vi "ADAM 5000 Get Data.vi"(11 "TCP Connection Refnum in":refnum<k5>) -> (1 "Voltages":dbl[](array[numeric])=[0.7972994999999994, -0.009129000000000609, -0.009129000000000609, -0.009585900000000258, -0.009129000000000609, -0.009585900000000258, -0.009585900000000258, -0.009585900000000258], 2 "TC Array":dbl[](array[numeric])=[21.380699999999997, 27.4835, 27.4835, 27.4835, 27.4835, 27.378999999999998, 27.4835], 3 "TCP Connection Refnum (dup)":refnum<k5>)   [LabVIEW 2018]
uses:
  nimodbus121/71/vi.lib/NI Modbus.llb/MB Modbus Command.ctl
panel:
  out "error out 2":errorcluster
  in  "Modbus Voltage Command":T1={"Function Code"=3, "Starting Address"=0, "Quantity"=8, "Data"=[], "Discrete"=[]} {"Function Code" items=["Read Coils"=1, "Read Discrete Inputs"=2, "Read Holding Registers"=3, "Read Input Registers"=4, "Write Single Coil"=5, "Write Single Register"=6, "Read Exception Status"=7, "Write Multiple Coils"=15, "Write Multiple Registers"=16]}
  out "Slave Input Registers 3":u16[](array[numeric])=[38065, 32770, 32770, 32767, 32770, 32767, 32767, 32767] caption="Slave Input Registers (Read Only)"
  out "error out":errorcluster
  in  "Modbus TC Command":T1={"Function Code"=3, "Starting Address"=16, "Quantity"=7, "Data"=[], "Discrete"=[]} {"Function Code" items=["Read Coils"=1, "Read Discrete Inputs"=2, "Read Holding Registers"=3, "Read Input Registers"=4, "Write Single Coil"=5, "Write Single Register"=6, "Read Exception Status"=7, "Write Multiple Coils"=15, "Write Multiple Registers"=16]}
  out "Slave Input Registers 2":u16[](array[numeric])=[1023, 1315, 1315, 1315, 1315, 1310, 1315] caption="Slave Input Registers (Read Only)"
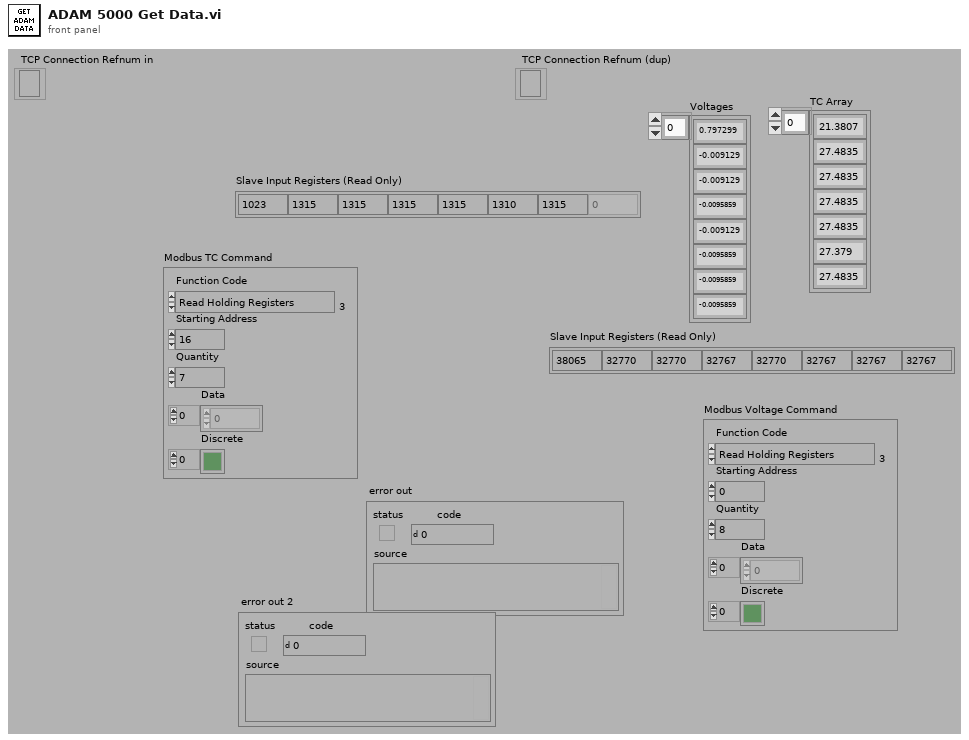
[diagram p1: front panel]
types:
  T1 = typedef "MB Modbus Command.ctl" = cluster{"Function Code":u8, "Starting Address":u16, "Quantity":u16, "Data":u16[], "Discrete":bool[]}
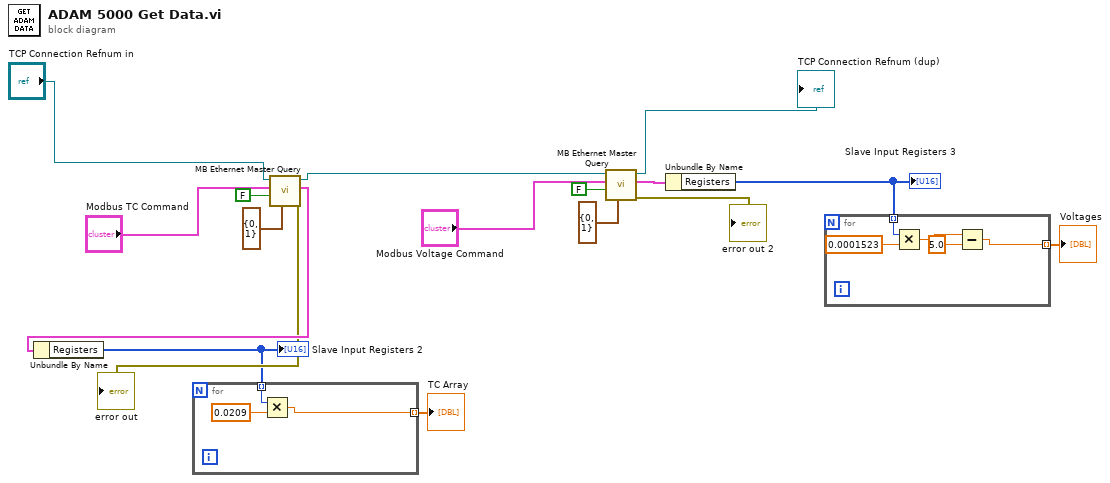
[diagram p0: block diagram]
diagram:
  n1 = call "MB Ethernet Master Query.vi"("MBAP Header"=cluster{"Transaction ID":u16, "Unit ID":u8} {"Transaction ID"=0, "Unit ID"=1}, "Use MODBUS Data Unit?"=FALSE, "Modbus Command"="Modbus TC Command", "TCP Connection Refnum in"="TCP Connection Refnum in") -> ("error out"=→"error out":errorcluster, "Registers"=w16:cluster{"Registers":u16[], "Discrete":bool[]}, "TCP Connection Refnum (dup)"=w3:refnum<k5>)  [unwired: 3 in, 2 out]
  n2 = Unbundle By Name(w16) -> ("Registers"=w12:u16[])
  "Slave Input Registers 2" <- w12
  n3 = for {
    tunnel: w12 -> [w20] mode=indexing
    tunnel: [w18] -> w11 mode=indexing
    n4 = Multiply(x=w20, y=0.0209) -> (x*y=w18:dbl)
  }
  "TC Array" <- w11
  n5 = call "MB Ethernet Master Query.vi"("MBAP Header"=cluster{"Transaction ID":u16, "Unit ID":u8} {"Transaction ID"=0, "Unit ID"=1}, "Use MODBUS Data Unit?"=FALSE, "Modbus Command"="Modbus Voltage Command", "TCP Connection Refnum in"=w3) -> ("error out"=→"error out 2":errorcluster, "Registers"=w9:cluster{"Registers":u16[], "Discrete":bool[]}, "TCP Connection Refnum (dup)"=→"TCP Connection Refnum (dup)":refnum<k5>)  [unwired: 3 in, 2 out]
  n6 = Unbundle By Name(w9) -> ("Registers"=w5:u16[])
  "Slave Input Registers 3" <- w5
  n7 = for {
    tunnel: w5 -> [w25] mode=indexing
    tunnel: [w21] -> w4 mode=indexing
    n8 = Multiply(x=w25, y=0.0001523) -> (x*y=w23:dbl)
    n9 = Subtract(x=w23, y=5.0) -> (x-y=w21:dbl)
  }
  "Voltages" <- w4
